vi "CropPortPos.vi"(11 "Position":dbl) -> (3 "New Position":dbl)   [LabVIEW 2015]
uses:
  Framework/Robot Global Data.vi
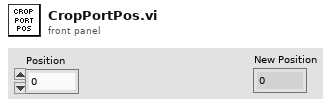
[diagram p1: front panel]
types:
  T1 = typedef "PortC Settings Type Def.ctl" = cluster{"PortC Down":dbl, "PortC Up":dbl, "Port Increments":dbl}
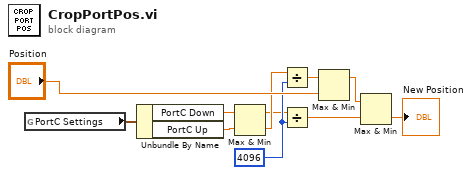
[diagram p0: block diagram]
diagram:
  w6 = 4096
  n1 = global read "Robot Global Data.vi" "PortC Settings"() -> (w5:T1)
  n2 = Unbundle By Name(w5) -> ("PortC Down"=w4:dbl, "PortC Up"=w2:dbl)
  n3 = Max & Min(x=w4, y=w2) -> (max(x,y)=w1:dbl, min(x,y)=w3:dbl)
  n4 = Divide(x=w3, y=w6) -> (x/y=w7:dbl)
  n5 = Divide(x=w1, y=w6) -> (x/y=w8:dbl)
  n6 = Max & Min(x=w7, y="Position") -> (max(x,y)=w10:dbl)  [unwired: 1 out]
  n7 = Max & Min(x=w10, y=w8) -> (min(x,y)=→"New Position":dbl)  [unwired: 1 out]
